vi "Status.vi"(8 "error in (no error)":errorcluster, 11 "Huber Settings In":T1) -> (0 "error out":errorcluster, 1 "Connection Error":bool, 2 "Running":bool, 3 "Huber Settings Out":T1, 4 "Temp":i32)   [LabVIEW 2021, in "Huber Ministat 230 TCU.lvlib"]
uses:
  Huber Ministat 230 TCU.lvlib
  Huber Settings.ctl
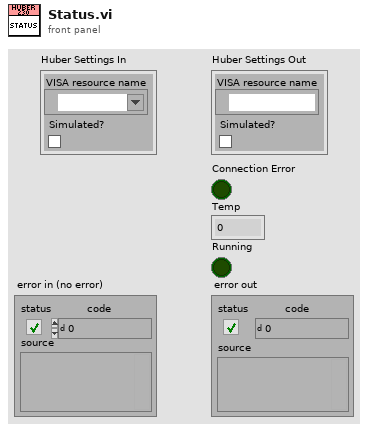
[diagram p1: front panel]
types:
  T1 = typedef "Huber Ministat 230 TCU.lvlib/Huber Settings.ctl" = cluster{"VISA resource name":refnum<visa-resource-name>, "Simulated?":bool}
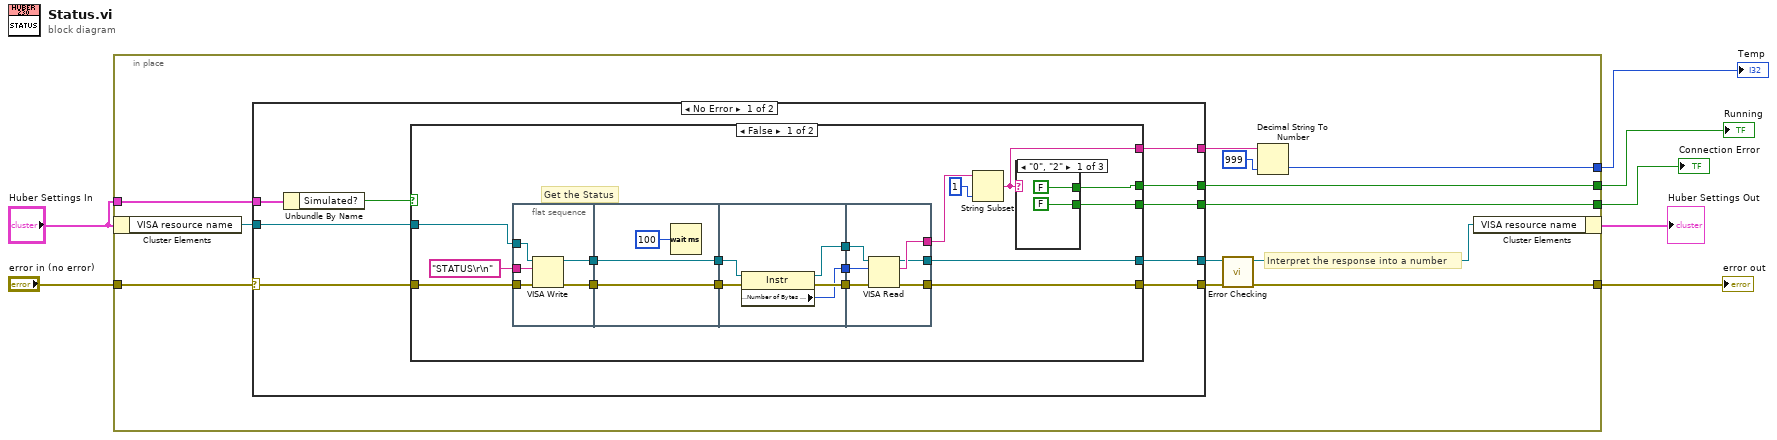
[diagram p0: block diagram]
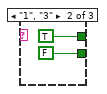
[diagram p2: hidden frame]
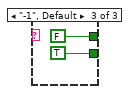
[diagram p3: hidden frame]
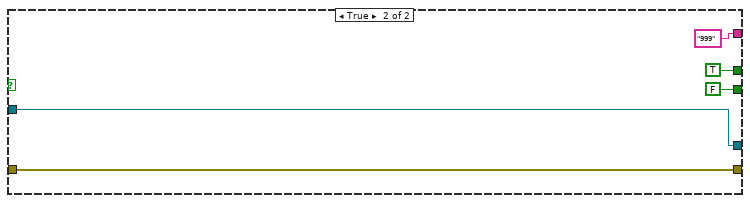
[diagram p4: hidden frame]
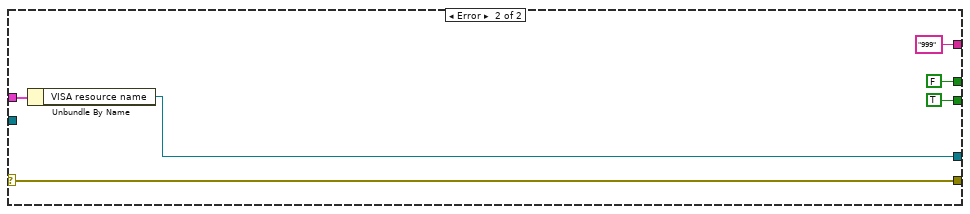
[diagram p5: hidden frame]
diagram:
  n1 = in-place {
    in-place-border: "error in (no error)" -> [w19]
    in-place-border: [w16] -> w6
    in-place-border: "Huber Settings In" -> [w15]
    in-place-border: [w10] -> w3
    in-place-border: [w9] -> w2
    in-place-border: [w8] -> w1
    # "Interpret the response into a number"
    n2 = in-place-cluster #1("Huber Settings In") -> ("VISA resource name"=w12:refnum<visa-resource-name>)
    n3 = case shown="No Error" w19 {
      selector: w19 -> [w28 w81]
      tunnel: w15 -> [w26 w80]
      tunnel: [w27 w81] -> w17
      tunnel: [w25 w79] -> w18
      tunnel: [w23 TRUE] -> w10
      tunnel: [w22 FALSE] -> w8
      tunnel: [w21 "999" ("read buffer")] -> w14
      tunnel: w12 -> [w20 _]
      frame No Error {
        n4 = Unbundle By Name(w26) -> ("Simulated?"=w24:bool)
        n5 = case shown="False" w24 {
          tunnel: w28 -> [w31 w75]
          tunnel: [w33 w75] -> w27
          tunnel: [w34 w74] -> w25
          tunnel: w20 -> [w32 w74]
          tunnel: [w42 FALSE] -> w23
          tunnel: [w30 TRUE] -> w22
          tunnel: [w29 "999" ("read buffer")] -> w21
          frame False {
            # "Get the Status"
            n6 = flat-sequence {
              tunnel: "STATUS\r\n" ("string") -> [w56]
              tunnel: [w55] -> w44
              tunnel: [w54] -> w43
              tunnel: w32 -> [w53]
              tunnel: w31 -> [w52]
              tunnel: w44 -> [w58]
              tunnel: w43 -> [w57]
              tunnel: [w58] -> w36
              tunnel: [w57] -> w35
              tunnel: [w62] -> w39
              tunnel: [w61] -> w38
              tunnel: [w60] -> w37
              tunnel: w36 -> [w64]
              tunnel: w35 -> [w63]
              tunnel: [w70] -> w33
              tunnel: [w69] -> w40
              tunnel: [w68] -> w34
              tunnel: w39 -> [w67]
              tunnel: w38 -> [w66]
              tunnel: w37 -> [w65]
              frame #0 {
                n7 = VISA Write(VISA resource name=w53, write buffer=w56, error in (no error)=w52) -> (VISA resource name out=w55:refnum<visa-resource-name>, error out=w54:errorcluster)  [unwired: 1 out]
              }
              frame #1 {
                n8 = Wait (ms)(milliseconds to wait=u32 100) -> ()  [unwired: 1 out]
              }
              frame #2 {
                n9 = property class="Instr"(reference=w64, error in=w63) -> (reference out=w62:refnum<visa-resource-name>, error out=w61:errorcluster, "Serial Settings:Number of Bytes at Serial Port"=w60:u32)
              }
              frame #3 {
                n10 = VISA Read(VISA resource name=w67, byte count=w65, error in (no error)=w66) -> (VISA resource name out=w68:refnum<visa-resource-name>, read buffer=w69:string, error out=w70:errorcluster)  [unwired: 1 out]
              }
            }
            n11 = String Subset(string=w40, length (rest)=1 ("length (rest)")) -> (substring=w29:string)  [unwired: 1 in]
            n12 = case shown="\"0\", \"2\"" w29 {
              tunnel: [FALSE FALSE TRUE] -> w42
              tunnel: [FALSE TRUE FALSE] -> w30
              frame "0", "2" {
              }
              frame "1", "3" {
              }
              frame "-1", Default {
              }
            }
          }
          frame True {
          }
        }
      }
      frame Error {
        n13 = Unbundle By Name(w80) -> ("VISA resource name"=w79:refnum<visa-resource-name>)
      }
    }
    n14 = call "Error Checking.vi"("error in (no error)"=w17, "VISA resource name"=w18) -> ("error out"=w16:errorcluster, "VISA resource name"=w11:refnum<visa-resource-name>)  [unwired: 7 in, 1 out]
    n15 = Decimal String To Number(string=w14, default (0L)=999 ("default (0 I32)")) -> (number=w9:i32)  [unwired: 1 in, 1 out]
    n16 = in-place-cluster #1("VISA resource name"=w11) -> (→"Huber Settings Out":T1)
  }
  "error out" <- w6
  "Connection Error" <- w3
  "Temp" <- w2
  "Running" <- w1
